vi "Reset.vi"(0 "VISA Resource Name":refnum<visa-resource-name>, 11 "error in (no error)":errorcluster) -> (4 "VISA Resource Name Out":refnum<visa-resource-name>, 15 "error out":errorcluster)   [LabVIEW 2018, in "Agilent 34970.lvlib"]
doc: "This VI resets the instrument, and then sends a set of default setup commands to the instrument. If a Reset command is not supported, it will return a warning."
uses:
  Agilent 34970.lvlib
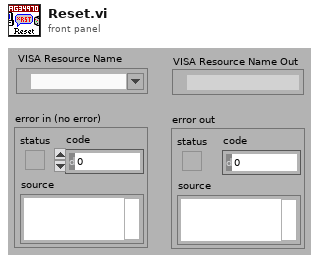
[diagram p1: front panel]
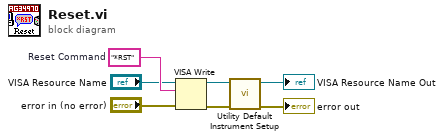
[diagram p0: block diagram]
diagram:
  w6 = "*RST"  # Reset Command
  n1 = VISA Write(VISA resource name="VISA Resource Name", write buffer=w6, error in (no error)="error in (no error)") -> (VISA resource name out=w2:refnum<visa-resource-name>, error out=w7:errorcluster)  [unwired: 1 out]
  n2 = call "Utility Default Instrument Setup.vi"("error in (no error)"=w7, "VISA Resource Name"=w2) -> ("error out"=→"error out":errorcluster, "VISA Resource Name Out"=→"VISA Resource Name Out":refnum<visa-resource-name>)  [unwired: 8 in]
